vi "do_povorota_kvaly.vi"() -> ()   [LabVIEW 2017]
uses:
  <vilib>/userdefined/High Color/IMAQdx.ctl
  <vilib>/vision/driver/NI_Vision_Acquisition_Software.lvlib
panel:
  out "X":sgl
  # "s"
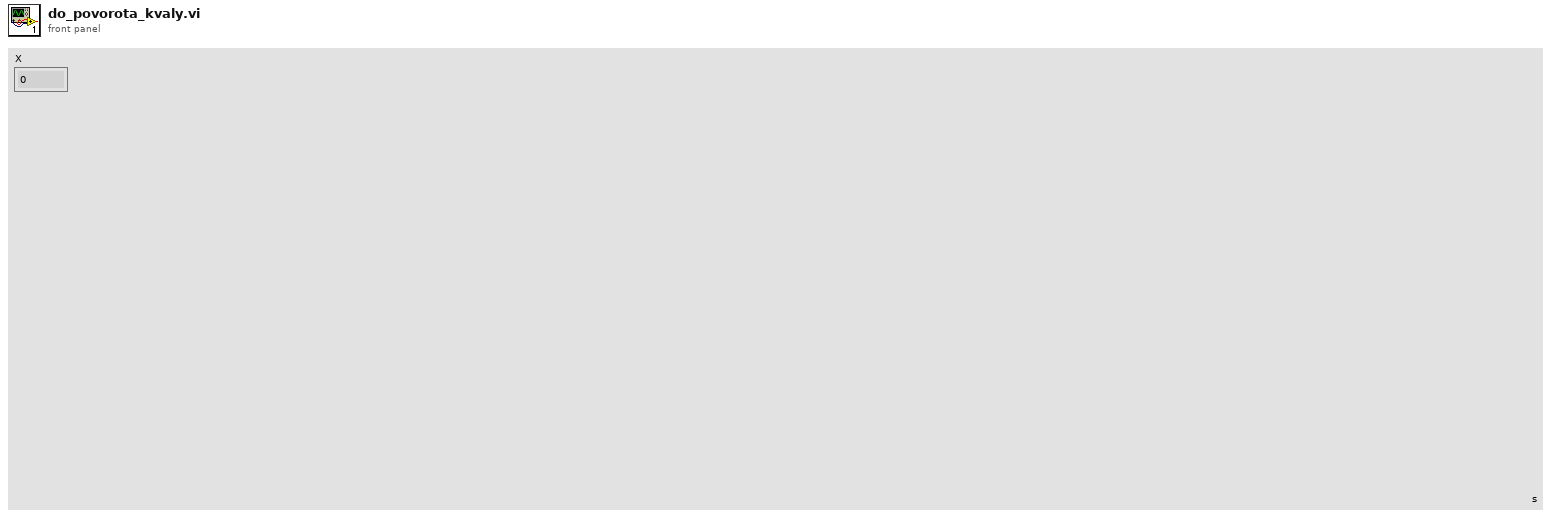
[diagram p1: front panel]
types:
  T1 = typedef "IMAQdx.ctl" = refnum<k21>
  T2 = typedef "IMAQ Image.ctl" = refnum<image>
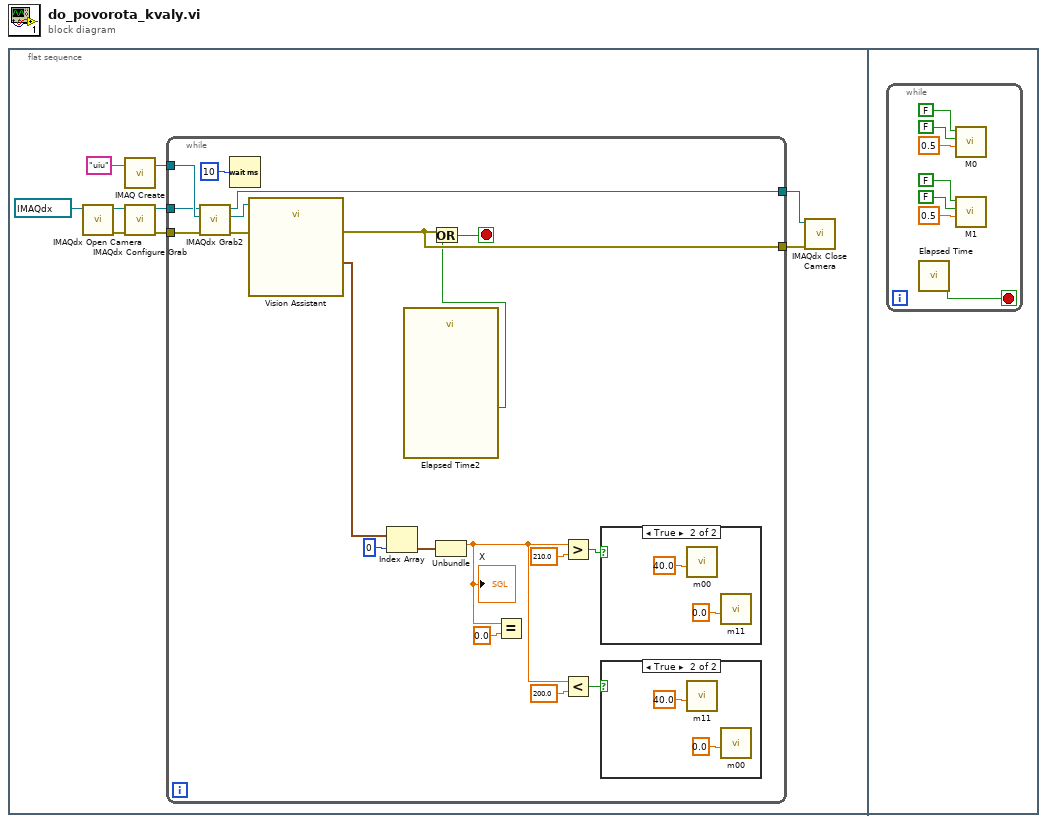
[diagram p0: block diagram]
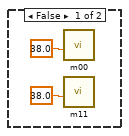
[diagram p2: hidden frame]
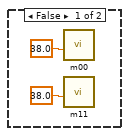
[diagram p3: hidden frame]
diagram:
  n1 = flat-sequence {
    frame #0 {
      n2 = call <vilib>:"IMAQdx Open Camera.vi"("Session In"=T1 "cam1") -> ("error out"=w6:errorcluster, "Session Out"=w5:T1)  [unwired: 9 in]
      n3 = call "IMAQ Create"("Image Name"="uiu") -> ("New Image"=w3:T2)  [unwired: 4 in, 1 out]
      n4 = call <vilib>:"IMAQdx Configure Grab.vi"("error in"=w6, "Session In"=w5) -> ("error out"=w7:errorcluster, "Session Out"=w4:T1)  [unwired: 8 in]
      n5 = while {
        tunnel: w7 -> [w23]
        tunnel: w3 -> [w22]
        tunnel: w4 -> [w21]
        tunnel: [w20] -> w9
        tunnel: [w18] -> w8
        stop <- w19 stop-if-true
        n6 = call <vilib>:"IMAQdx Grab2.vi"("error in"=w23, "Image In"=w22, "Session In"=w21) -> ("error out"=w25:errorcluster, "Image Out"=w24:T2, "Session Out"=w20:T1)  [unwired: 5 in, 1 out]
        n7 = Wait (ms)(milliseconds to wait=u32 10) -> ()  [unwired: 1 out]
        n8 = call "Vision Assistant"("Image In"=w24, "error in"=w25) -> ("Edges Coordinates (Edge Detector 1)"=w28:cluster{"X":sgl, "Y":sgl}[], "error out"=w18:errorcluster)  [unwired: 22 in, 2 out]
        n9 = Index Array(array=w28, index=0) -> (element=w27:cluster{"X":sgl, "Y":sgl})
        n10 = call "Elapsed Time2"() -> ("Time has Elapsed"=w10:bool)  [unwired: 12 in, 7 out]
        n11 = Or(x=w18, y=w10) -> (x .or. y?=w19:bool)
        n12 = Unbundle(w27) -> ("X"=w13:sgl)  [unwired: 1 out]
        "X" <- w13
        n13 = Equal?(x=w13, y=sgl 0.0) -> ()  [unwired: 1 out]
        n14 = Greater?(x=w13, y=sgl 210.0) -> (0:w16:bool)
        n15 = Less?(x=w13, y=sgl 200.0) -> (x < y?=w12:bool)
        n16 = case shown="True" w16 {
          frame False {
            n17 = call "m00.vi"("position"=38.0) -> ()  [unwired: 10 in, 1 out]
            n18 = call "m11.vi"("position"=38.0) -> ()  [unwired: 10 in, 1 out]
          }
          frame True {
            n19 = call "m00.vi"("position"=40.0) -> ()  [unwired: 10 in, 1 out]
            n20 = call "m11.vi"("position"=0.0) -> ()  [unwired: 10 in, 1 out]
          }
        }
        n21 = case shown="True" w12 {
          frame False {
            n22 = call "m00.vi"("position"=38.0) -> ()  [unwired: 10 in, 1 out]
            n23 = call "m11.vi"("position"=38.0) -> ()  [unwired: 10 in, 1 out]
          }
          frame True {
            n24 = call "m11.vi"("position"=40.0) -> ()  [unwired: 10 in, 1 out]
            n25 = call "m00.vi"("position"=0.0) -> ()  [unwired: 10 in, 1 out]
          }
        }
      }
      n26 = call <vilib>:"IMAQdx Close Camera.vi"("error in"=w8, "Session In"=w9) -> ()  [unwired: 9 in, 1 out]
    }
    frame #1 {
      n27 = while {
        stop <- w43 stop-if-true
        n28 = call "Elapsed Time"() -> ("Time has Elapsed"=w43:bool)  [unwired: 12 in, 7 out]
        n29 = call "M0.vi"("Duty Cycle"=0.5, "назад"=FALSE ("вперед"), "вперед"=FALSE ("назад")) -> ()  [unwired: 8 in, 1 out]
        n30 = call "M1.vi"("Duty Cycle"=0.5, "назад"=FALSE ("вперед"), "вперед"=FALSE ("назад")) -> ()  [unwired: 8 in, 1 out]
      }
    }
  }
